vi "ejer5 - copia.vi"() -> ()   [LabVIEW 2014]
panel:
  in  "Tab Control":T1(tab)
  in  "Frecuencia":dbl(knob) scale=0.0..100.0
  in  "Amplitud":dbl(knob) scale=0.0..100.0
  out "Waveform Chart":dynamicdata(graph)
  out "Aleaorio":dbl[](array[numeric])
  out "Cantidad de números generados":i32
  out "PRIMO":dbl[](array[numeric]) caption="Primos"
  out "Cantidad de números primos":i32
  out "Pares":dbl[](array[numeric])
  out "Impar":dbl[](array[numeric])
  out "Cantidad de números pares":i32
  out "Cantidad de números impares":i32
  out "Mensaje Final":string
  in  "Número del mes de nacimiento":dbl
  in  "Año de nacimiento":dbl
  in  "Nombre y Apellido":string
  out "Matriz Trapuesta":dbl[][](array[numeric])
  out "Matriz Original":dbl[][](array[numeric])
  out "Máximos":dbl[](array[numeric])
  out "Mínimos":dbl[](array[numeric])
  in  "STOP":bool
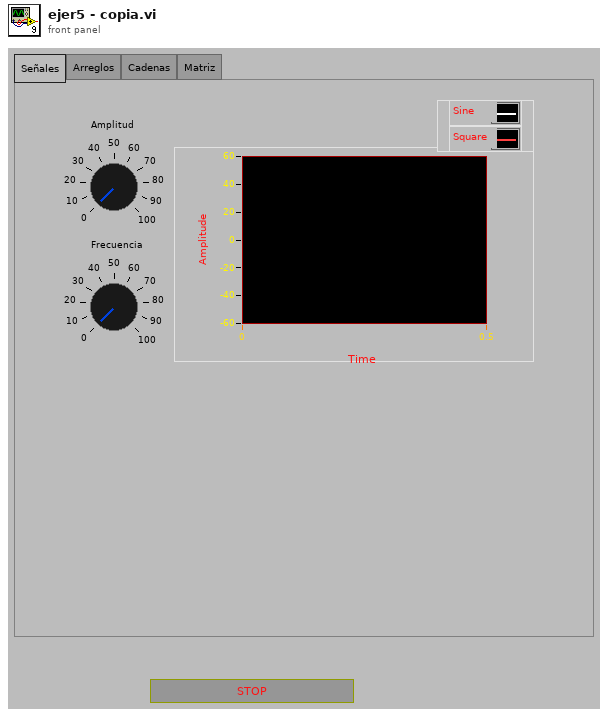
[diagram p1: front panel]
types:
  T1 = enum32{"Señales", "Arreglos", "Cadenas", "Matriz"}
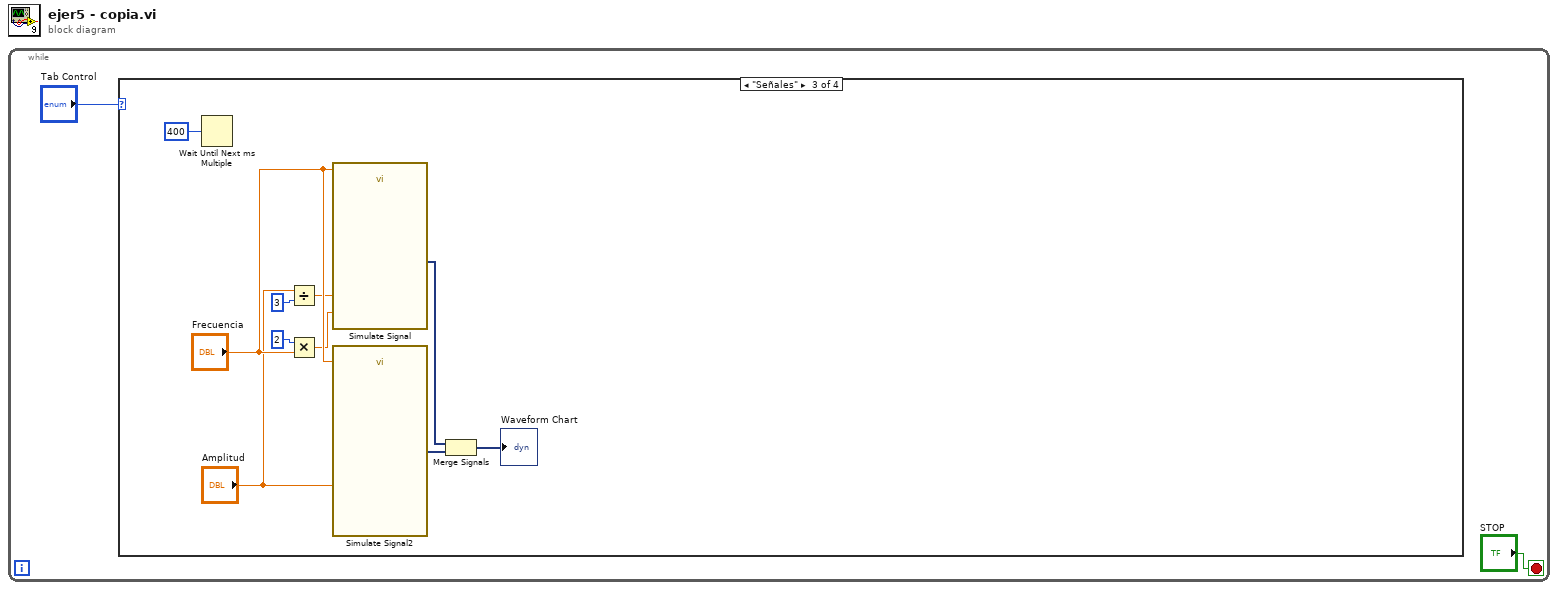
[diagram p0: block diagram]
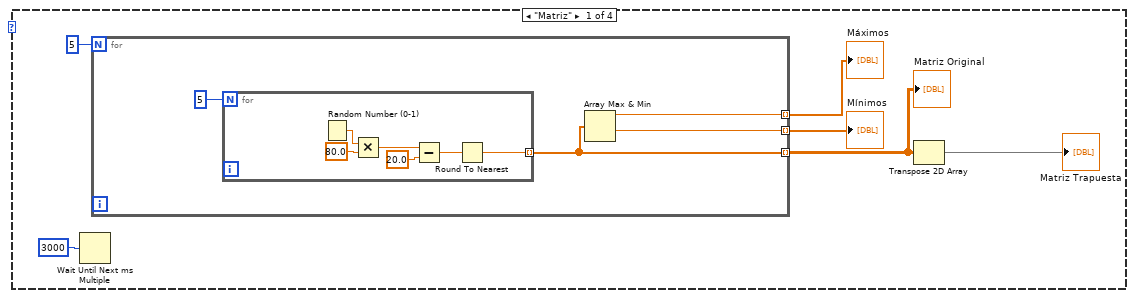
[diagram p2: hidden frame]
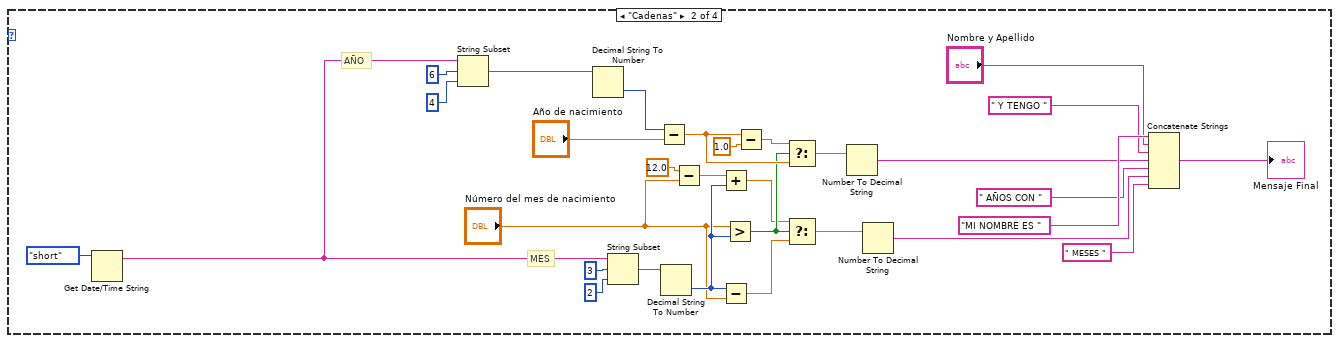
[diagram p3: hidden frame]
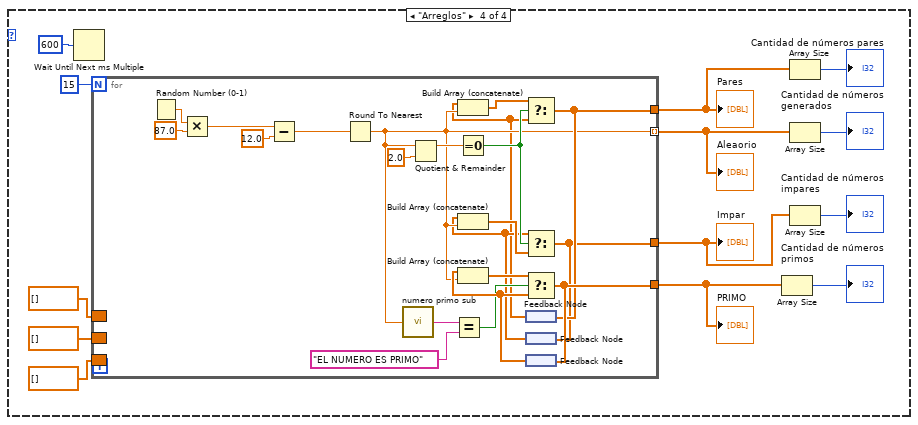
[diagram p4: hidden frame]
diagram:
  n1 = while {
    stop <- "STOP" stop-if-true
    n2 = case shown="\"Señales\"" "Tab Control" {
      frame "Matriz" {
        n3 = Wait Until Next ms Multiple(millisecond multiple=u32 3000) -> ()  [unwired: 1 out]
        n4 = for {
          N: 5 -> [_]
          tunnel: [w11] -> w6 mode=indexing
          tunnel: [w10] -> w4 mode=indexing
          tunnel: [w9] -> w3 mode=indexing
          n5 = for {
            N: 5 -> [_]
            tunnel: [w14] -> w11 mode=indexing
            n6 = Random Number (0-1)() -> (number: 0 to 1=w18:dbl)
            n7 = Multiply(x=w18, y=80.0) -> (x*y=w13:dbl)
            n8 = Subtract(x=w13, y=20.0) -> (x-y=w15:dbl)
            n9 = Round To Nearest(number=w15) -> (nearest integer value=w14:dbl)
          }
          n10 = Array Max & Min(array=w11) -> (max value=w10:dbl, min value=w9:dbl)  [unwired: 2 out]
        }
        "Matriz Original" <- w6
        "Máximos" <- w4
        "Mínimos" <- w3
        n11 = Transpose 2D Array(2D array=w6) -> (transposed array=→"Matriz Trapuesta":dbl[][])
      }
      frame "Cadenas" {
        # "AÑO"
        # "MES"
        n12 = Get Date/Time String(date format (0)=enum16{"short", "long", "abbreviated"}."short") -> (date string=w23:string)  [unwired: 2 in, 1 out]
        n13 = String Subset(string=w23, offset (0)=6, length (rest)=4 ("length (rest)")) -> (substring=w38:string)
        n14 = Decimal String To Number(string=w38) -> (number=w21:i32)  [unwired: 2 in, 1 out]
        n15 = String Subset(string=w23, offset (0)=3, length (rest)=2 ("length (rest)")) -> (substring=w41:string)
        n16 = Subtract(x=w21, y="Año de nacimiento") -> (x-y=w35:dbl)
        n17 = Decimal String To Number(string=w41) -> (number=w28:i32)  [unwired: 2 in, 1 out]
        n18 = Subtract(x=12.0, y="Número del mes de nacimiento") -> (x-y=w29:dbl)
        n19 = Add(x=w29, y=w28) -> (x+y=w19:dbl)
        n20 = Subtract(x=w28, y="Número del mes de nacimiento") -> (x-y=w27:dbl)
        n21 = Greater?(x="Número del mes de nacimiento", y=w28) -> (0:w31:bool)
        n22 = Subtract(x=w35, y=1.0) -> (x-y=w36:dbl)
        n23 = Select(t=w36, s=w31, f=w35) -> (s? t:f=w34:dbl)
        n24 = Select(t=w19, s=w31, f=w27) -> (s? t:f=w26:dbl)
        n25 = Number To Decimal String(number=w34) -> (decimal integer string=w33:string)  [unwired: 1 in]
        n26 = Number To Decimal String(number=w26) -> (decimal integer string=w25:string)  [unwired: 1 in]
        n27 = Concatenate Strings "Concatenate Strings"("MI NOMBRE ES " ("string"), "Nombre y Apellido", " Y TENGO " ("string"), w33, " AÑOS CON " ("string"), w25, " MESES " ("string")) -> (→"Mensaje Final":string)
      }
      frame "Señales" {
        n28 = Wait Until Next ms Multiple(millisecond multiple=u32 400) -> ()  [unwired: 1 out]
        n29 = Divide(x="Amplitud", y=3) -> (x/y=w49:dbl)
        n30 = Multiply(x=2, y="Frecuencia") -> (x*y=w52:dbl)
        n31 = call "Simulate Signal"("Offset"="Frecuencia", "Frequency"=w52, "Amplitude"=w49) -> ("Sine"=w55:dynamicdata)  [unwired: 11 in, 1 out]
        n32 = call "Simulate Signal2"("Frequency"="Frecuencia", "Amplitude"="Amplitud") -> ("Square"=w58:dynamicdata)  [unwired: 12 in, 1 out]
        n33 = Merge Signals(w55, w58) -> (→"Waveform Chart":dynamicdata)
      }
      frame "Arreglos" {
        n34 = Wait Until Next ms Multiple(millisecond multiple=u32 600) -> ()  [unwired: 1 out]
        n35 = for {
          N: 15 -> [_]
          tunnel: [w74] -> w59 mode=indexing
          tunnel: [w86] -> w68
          tunnel: [w83] -> w64
          tunnel: [w78] -> w62
          border: dbl[] [] -> [_]
          border: dbl[] [] -> [_]
          border: dbl[] [] -> [_]
          n36 = Random Number (0-1)() -> (number: 0 to 1=w92:dbl)
          n37 = Multiply(x=w92, y=87.0) -> (x*y=w90:dbl)
          n38 = Subtract(x=w90, y=12.0 ("x*y")) -> (x-y=w85:dbl)
          n39 = Round To Nearest(number=w85) -> (nearest integer value=w74:dbl)
          n40 = call "numero primo sub.vi"("INGRESAR EL NUMERO"=w74) -> (0:w81:string)
          n41 = Quotient & Remainder(x=w74, y=2.0) -> (x-y*floor(x/y)=w80:dbl)  [unwired: 1 out]
          n42 = Equal?(x=w81, y="EL NUMERO ES PRIMO") -> (x = y?=w75:bool)
          n43 = Equal To 0?(x=w80) -> (x = 0?=w82:bool)
          n44 = feedback #1() -> (w72:dbl[])
          n45 = Build Array (concatenate)(w72, w74) -> (w76:dbl[])
          n46 = Select(t=w76, s=w82, f=w72) -> (s? t:f=w83:dbl[])
          n47 = feedback-in #1(w83) -> ()
          n48 = feedback #2() -> (w73:dbl[])
          n49 = Build Array (concatenate)(w73, w74) -> (w79:dbl[])
          n50 = Select(t=w73, s=w82, f=w79) -> (s? t:f=w78:dbl[])
          n51 = feedback-in #2(w78) -> ()
          n52 = feedback #3() -> (w87:dbl[])
          n53 = Build Array (concatenate)(w87, w74) -> (w77:dbl[])
          n54 = Select(t=w77, s=w75, f=w87) -> (s? t:f=w86:dbl[])
          n55 = feedback-in #3(w86) -> ()
        }
        "Aleaorio" <- w59
        "PRIMO" <- w68
        "Pares" <- w64
        "Impar" <- w62
        n56 = Array Size(array=w68) -> (size(s)=→"Cantidad de números primos":i32)
        n57 = Array Size(array=w64) -> (size(s)=→"Cantidad de números pares":i32)
        n58 = Array Size(array=w59) -> (size(s)=→"Cantidad de números generados":i32)
        n59 = Array Size(array=w62) -> (size(s)=→"Cantidad de números impares":i32)
      }
    }
  }
